vi "S2C_FORNAX_Proc_CmdStatusMsg.vi"(8 "Error In":errorcluster, 10 "CmdMsg":string, 11 "CmdString":string) -> (0 "Error Out":errorcluster, 3 "StatusMsg":string)   [LabVIEW 2015]
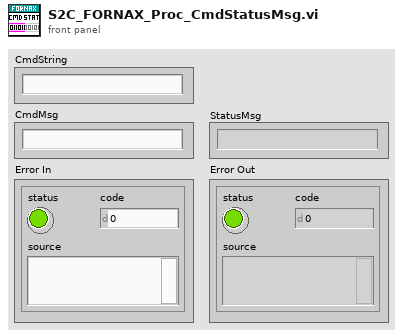
[diagram p1: front panel]
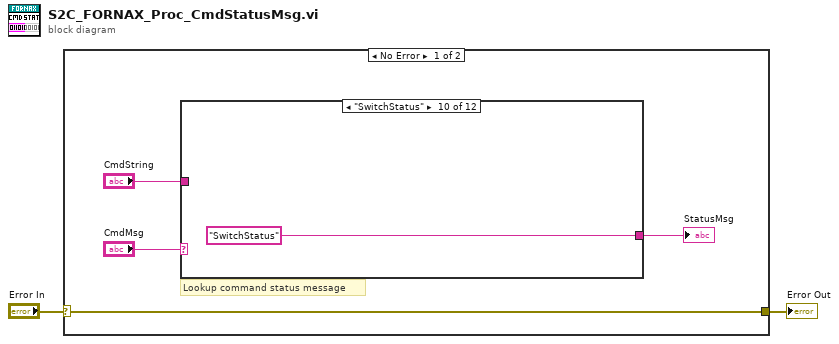
[diagram p0: block diagram]
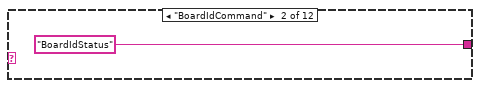
[diagram p3: hidden frame]
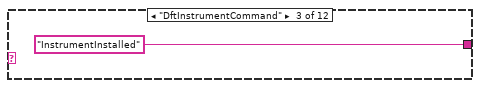
[diagram p4: hidden frame]
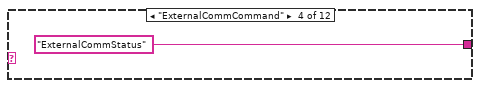
[diagram p5: hidden frame]
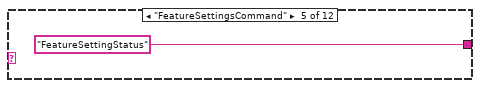
[diagram p6: hidden frame]
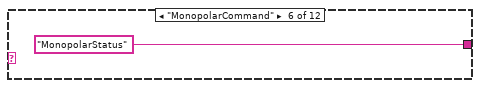
[diagram p7: hidden frame]
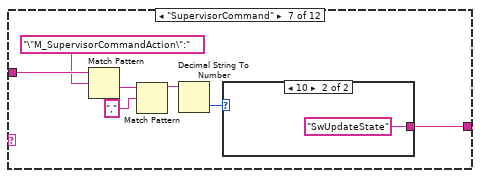
[diagram p8: hidden frame]
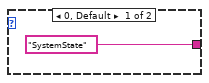
[diagram p9: hidden frame]
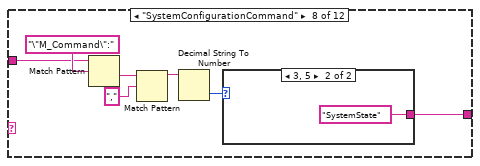
[diagram p10: hidden frame]
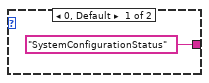
[diagram p11: hidden frame]
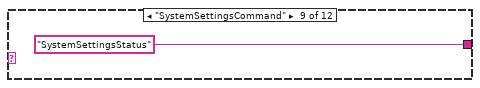
[diagram p12: hidden frame]
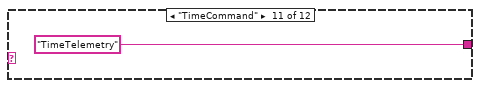
[diagram p13: hidden frame]
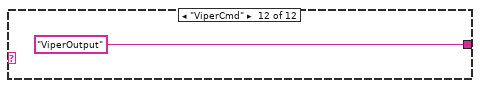
[diagram p14: hidden frame]
diagram:
  n1 = case shown="No Error" "Error In" {
    selector: "Error In" -> [w6 w34]
    tunnel: [w6 w34] -> w1
    frame No Error {
      # "Lookup command status message"
      n2 = case shown="\"SwitchStatus\"" "CmdMsg" {
        tunnel: [_ "BoardIdStatus" "InstrumentInstalled" "ExternalCommStatus" "FeatureSettingStatus" "MonopolarStatus" w13 w21 "SystemSettingsStatus" "SwitchStatus" "TimeTelemetry" "ViperOutput"] -> w4
        tunnel: "CmdString" -> [_ _ _ _ _ _ w16 w24 _ _ _ _]
        frame "Unknown", Default {
        }
        frame "BoardIdCommand" {
        }
        frame "DftInstrumentCommand" {
        }
        frame "ExternalCommCommand" {
        }
        frame "FeatureSettingsCommand" {
        }
        frame "MonopolarCommand" {
        }
        frame "SupervisorCommand" {
          n3 = Match Pattern(string=w16, regular expression="\"M_SupervisorCommandAction\":") -> (after substring=w18:string)  [unwired: 1 in, 3 out]
          n4 = Match Pattern(string=w18, regular expression=",") -> (before substring=w15:string)  [unwired: 1 in, 3 out]
          n5 = Decimal String To Number(string=w15) -> (number=w14:i32)  [unwired: 2 in, 1 out]
          n6 = case shown="10" w14 {
            tunnel: ["SystemState" "SwUpdateState"] -> w13
            frame 0, Default {
            }
            frame 10 {
            }
          }
        }
        frame "SystemConfigurationCommand" {
          n7 = Match Pattern(string=w24, regular expression="\"M_Command\":") -> (after substring=w26:string)  [unwired: 1 in, 3 out]
          n8 = Match Pattern(string=w26, regular expression=",") -> (before substring=w23:string)  [unwired: 1 in, 3 out]
          n9 = Decimal String To Number(string=w23) -> (number=w22:i32)  [unwired: 2 in, 1 out]
          n10 = case shown="3, 5" w22 {
            tunnel: ["SystemConfigurationStatus" "SystemState"] -> w21
            frame 0, Default {
            }
            frame 3, 5 {
            }
          }
        }
        frame "SystemSettingsCommand" {
        }
        frame "SwitchStatus" {
        }
        frame "TimeCommand" {
        }
        frame "ViperCmd" {
        }
      }
      "StatusMsg" <- w4
    }
    frame Error {
    }
  }
  "Error Out" <- w1
